vi "Set DDG Lite Pulses Per Exposure.vi"(8 "error in (no error)":errorcluster, 10 "ui32Pulses":u32, 11 "channel":u32(ring)=65535 items=["AT_DDGLite_ChannelA"=1073741824, "AT_DDGLite_ChannelB"=1073741825, "AT_DDGLite_ChannelC"=1073741826]) -> (0 "error out":errorcluster, 3 "function return":u32)   [LabVIEW 2014, in "atmcd32d.lvlib"]
doc: "unsigned int WINAPI SetDDGLitePulsesPerExposure(AT_DDGLiteChannelId channel, at_u32 ui32Pulses);"
uses:
  atmcd32d.lvlib
  atmcd32d.dll
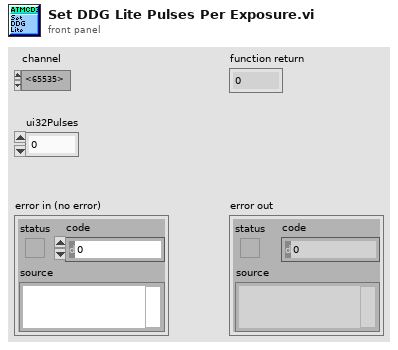
[diagram p1: front panel]
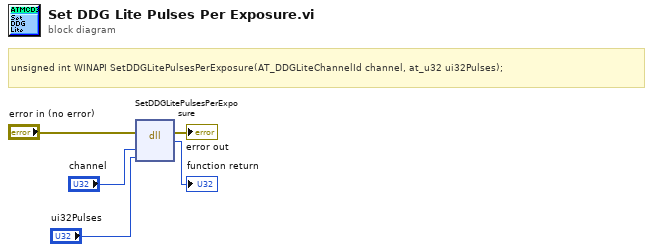
[diagram p0: block diagram]
diagram:
  # "unsigned int WINAPI SetDDGLitePulsesPerExposure(AT_DDGLiteChannelId channel, at_u32 ui32Pulses);"
  n1 = dll-call lib="C:/Users/Bakir/Documents/Lambda2-Testing/lib/Andorlib/atmcd32d.*" fn="SetDDGLitePulsesPerExposure"(error in="error in (no error)", "channel"="channel", "ui32Pulses"="ui32Pulses") -> (error out=→"error out":errorcluster, →"function return":u32)  [unwired: 4 in, 1 out]
